vi "get_config_cluster.vi"(8 "error in (no error)":errorcluster, 11 "TrajectoryDL110420DoubleCircle.lvclass in":refnum<class "TrajectoryDL110420DoubleCircle.lvclass">) -> (0 "error out":errorcluster, 2 "config cluster (variant)":variant, 3 "TrajectoryDL110420DoubleCircle.lvclass out":refnum<class "TrajectoryDL110420DoubleCircle.lvclass">)   [LabVIEW 2010, in "TrajectoryDL110420DoubleCircle.lvclass"]
uses:
  TrajectoryDL110420DoubleCircle.lvclass
  TrajectoryDL110420DoubleCircle.lvclass/TrajectoryDL110420DoubleCircle.ctl
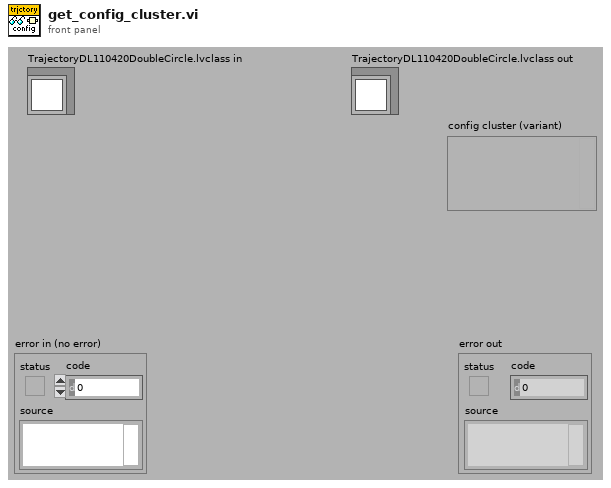
[diagram p1: front panel]
types:
  T1 = typedef "TrajectoryDL110420DoubleCircle.lvclass/config_data_cluster.ctl" = cluster{"xpaths":cluster{"x offset":string, "y offset":string, "z offset":string}}
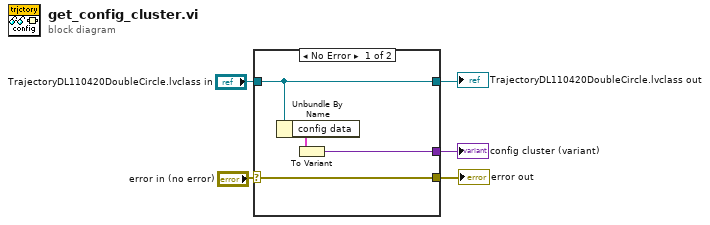
[diagram p0: block diagram]
diagram:
  n1 = case shown="No Error" "error in (no error)" {
    selector: "error in (no error)" -> [w7 w10]
    tunnel: "TrajectoryDL110420DoubleCircle.lvclass in" -> [w6 w11]
    tunnel: [w8 _] -> w5
    tunnel: [w7 w10] -> w3
    tunnel: [w6 w11] -> w1
    frame No Error {
      n2 = Unbundle By Name(w6) -> ("config data"=w9:T1)
      n3 = To Variant(anything=w9) -> (Variant=w8:variant)
    }
    frame Error {
    }
  }
  "error out" <- w3
  "config cluster (variant)" <- w5
  "TrajectoryDL110420DoubleCircle.lvclass out" <- w1
